vi "SendToDb.vi"(8 "error in (no error)":errorcluster, 11 "AnalogComparator in":refnum<class "AnalogComparator.lvclass">) -> (0 "error out":errorcluster, 3 "AnalogComparator out":refnum<class "AnalogComparator.lvclass">)   [LabVIEW 2019, in "AnalogComparator.lvclass"]
uses:
  AnalogComparator.lvclass
  D:/GIT H4000/H4000/src/Proccess_class/Proccess.lvclass
  Logger_class/EventData.ctl
  TypeDef/AlarmType.ctl
  Proccess_class/Proccess.lvclass/Proccess.ctl
  AnalogComparator.lvclass/AnalogComparator.ctl
  Logger_class/Logger.lvclass
  Proccess_class/Proccess.lvclass
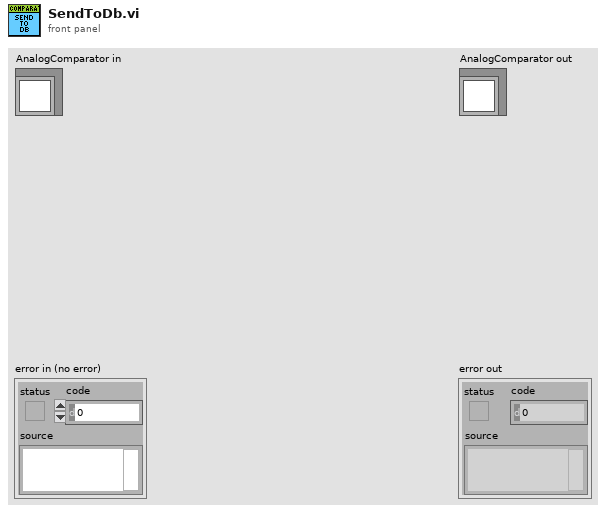
[diagram p1: front panel]
types:
  T1 = typedef "AlarmType.ctl" = enum16{"Normal", "Warning", "Alarm"}
  T2 = typedef "Logger.lvclass/EventData.ctl" = cluster{"obj_tag":string, "event_tag":string, "Description":string, "ALARM TYPE":T1, "Value DBL":dbl, "Value INT":i32, "Value STR":string, "Time Stamp":timestamp}
  T3 = typedef "Proccess.lvclass/TAGs.ctl" = cluster{"TAG":string, "PTAG":string, "DESC":string}
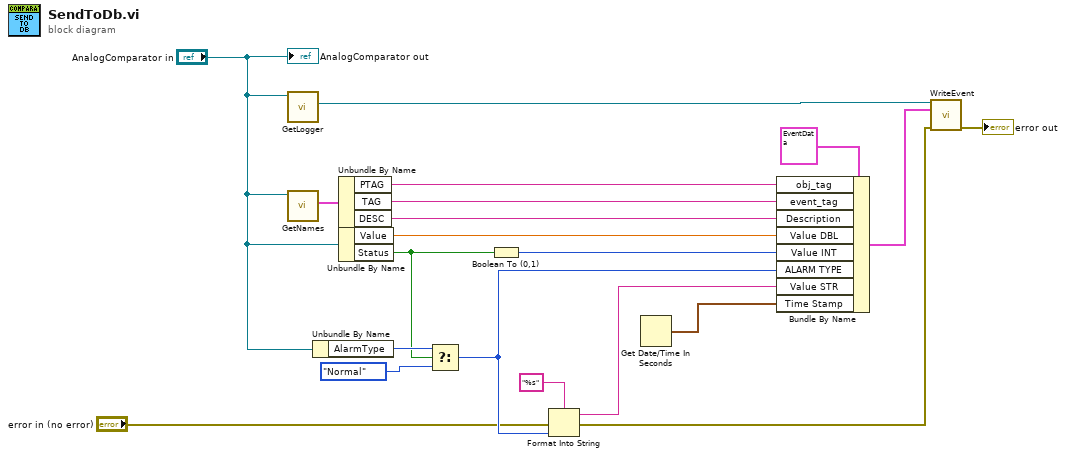
[diagram p0: block diagram]
diagram:
  n1 = call "GetLogger.vi"("Proccess in"="AnalogComparator in") -> ("Logger"=w18:refnum<class "Logger.lvclass">)  [unwired: 10 in]
  n2 = call "GetNames.vi"("Proccess in"="AnalogComparator in") -> ("Tags"=w17:T3)  [unwired: 10 in]
  n3 = Unbundle By Name("AnalogComparator in") -> ("AlarmType"=w10:T1)
  n4 = Unbundle By Name(w17) -> ("PTAG"=w15:string, "TAG"=w14:string, "DESC"=w13:string)
  n5 = Unbundle By Name("AnalogComparator in") -> ("Value"=w12:dbl, "Status"=w9:bool)
  n6 = Select(t=w10, s=w9, f=AlarmType."Normal") -> (s? t:f=w5:T1)
  n7 = Boolean To (0,1)(Boolean=w9) -> (0, 1=w11:i16)
  n8 = Format Into String(format string="%s", error in="error in (no error)", w5) -> (resulting string=w6:string, error out=w1:errorcluster)  [unwired: 1 in]
  n9 = Get Date/Time In Seconds() -> (seconds since 1Jan1904=w4:timestamp)
  n10 = Bundle By Name(cluster=T2 {"obj_tag"="", "event_tag"="", "Description"="", "ALARM TYPE"=enum."Alarm", "Value DBL"=0.0, "Value INT"=0, "Value STR"="", "Time Stamp"=timestamp(0 s since 1904-01-01)} ("Event"), "obj_tag"=w15, "event_tag"=w14, "Description"=w13, "Value DBL"=w12, "Value INT"=w11, "ALARM TYPE"=w5, "Value STR"=w6, "Time Stamp"=w4) -> (w2:T2)
  n11 = call "WriteEvent.vi"("reference in"=w18, "Event"=w2, "error in (no error)"=w1) -> ("error out"=→"error out":errorcluster)  [unwired: 11 in, 1 out]
  "AnalogComparator out" <- "AnalogComparator in"
